vi "Teste.vi"() -> ()   [LabVIEW 2020]
uses:
  C:/Users/Opto/Downloads/GrabTestTDNI/GrabFrame2.dll
  Downloads/GrabTestTDNI/GrabFrame2.dll
  C:/Users/Opto/Desktop/Equipamentos/Teste/DALSA.SaperaLT.SapClassBasic.dll
  DALSA.SaperaLT.SapClassBasic.dll
panel:
  out "error SaveFrame":errorcluster
  out "error final":errorcluster
  out "error sapTransfer Dispose":errorcluster
  out "countFrame":i32
  out "Wait":bool
  out "Destroy":bool
  out "Create":bool
  out "framesArr":i16[][](array[numeric])
  out "Abriu arquivo?":bool
  out "filePath":string="C:\\temp\\IC-47_TDI.ccf"
  # "Buffer"
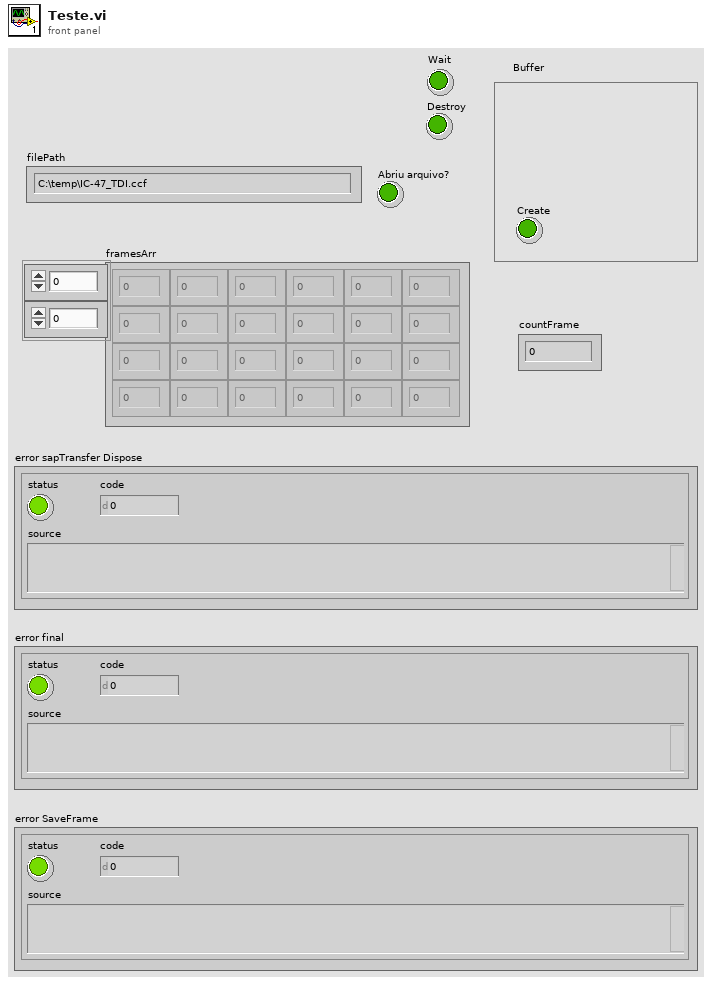
[diagram p1: front panel]
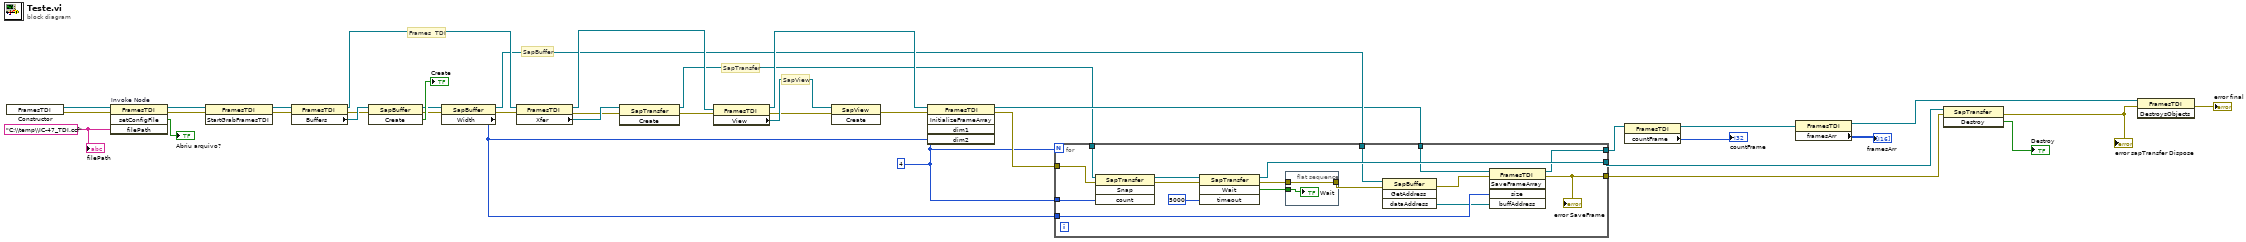
[diagram p0: block diagram]
diagram:
  w13 = 4 ("count")
  w35 = "C:\\temp\\IC-47_TDI.ccf" ("filePath")
  # "SapView"
  # "SapTransfer"
  # "SapBuffer"
  # "Frames  TDI"
  n1 = constructor class="FramesTDI"() -> (reference out=w38:refnum<k24>, error out=w39:errorcluster)  [unwired: 3 in, 1 out]
  n2 = invoke on="Invoke Node" class="FramesTDI" method="setConfigFile"(reference=w38, error in=w39, "filePath"=w35) -> (reference out=w37:refnum<k24>, error out=w36:errorcluster, "setConfigFile"=→"Abriu arquivo?":bool)  [unwired: 1 in, 1 out]
  n3 = invoke class="FramesTDI" method="StartGrabFramesTDI"(reference=w37, error in=w36) -> (reference out=w33:refnum<k24>, error out=w27:errorcluster)  [unwired: 1 in, 1 out]
  n4 = property class="FramesTDI"(reference=w33, error in=w27) -> (reference out=w20:refnum<k24>, error out=w26:errorcluster, "Buffers"=w32:refnum<k24>)
  n5 = invoke class="SapBuffer" method="Create"(reference=w32, error in=w26) -> (reference out=w28:refnum<k24>, error out=w25:errorcluster, "Create"=→"Create":bool)  [unwired: 1 in]
  n6 = property class="SapBuffer"(reference=w28, error in=w25) -> (reference out=w11:refnum<k24>, error out=w24:errorcluster, "Width"=w9:i32)
  n7 = property class="FramesTDI"(reference=w20, error in=w24) -> (reference out=w18:refnum<k24>, error out=w23:errorcluster, "Xfer"=w31:refnum<k24>)
  n8 = invoke class="SapTransfer" method="Create"(reference=w31, error in=w23) -> (reference out=w4:refnum<k24>, error out=w22:errorcluster)  [unwired: 1 in, 1 out]
  n9 = property class="FramesTDI"(reference=w18, error in=w22) -> (reference out=w17:refnum<k24>, error out=w21:errorcluster, "View"=w30:refnum<k24>)
  n10 = invoke class="SapView" method="Create"(reference=w30, error in=w21) -> (error out=w19:errorcluster)  [unwired: 1 in, 2 out]
  n11 = invoke class="FramesTDI" method="InitializeFrameArray"(reference=w17, error in=w19, "dim1"=w13, "dim2"=w9) -> (reference out=w10:refnum<k24>, error out=w14:errorcluster)  [unwired: 1 in, 3 out]
  n12 = for {
    N: w13 -> [_]
    tunnel: w4 -> [w56]
    tunnel: w14 -> [w55]
    tunnel: w13 -> [w54]
    tunnel: [w51] -> w12
    tunnel: w11 -> [w47]
    tunnel: w10 -> [w45]
    tunnel: w9 -> [w43]
    tunnel: [w41] -> w6
    tunnel: [w40] -> w8
    n13 = invoke class="SapTransfer" method="Snap"(reference=w56, error in=w55, "count"=w54) -> (reference out=w53:refnum<k24>, error out=w52:errorcluster)  [unwired: 1 in, 2 out]
    n14 = invoke class="SapTransfer" method="Wait"(reference=w53, error in=w52, "timeout"=5000) -> (reference out=w51:refnum<k24>, error out=w48:errorcluster, "Wait"=w49:bool)  [unwired: 1 in, 1 out]
    n15 = flat-sequence {
      tunnel: w49 -> [w58]
      tunnel: w48 -> [w57]
      tunnel: [w57] -> w46
      frame #0 {
        "Wait" <- w58
      }
    }
    n16 = invoke class="SapBuffer" method="GetAddress"(reference=w47, error in=w46) -> (error out=w44:errorcluster, "dataAddress"=w42:refnum<k24>)  [unwired: 2 in, 2 out]
    n17 = invoke class="FramesTDI" method="SaveFrameArray"(reference=w45, error in=w44, "size"=w43, "buffAddress"=w42) -> (reference out=w41:refnum<k24>, error out=w40:errorcluster)  [unwired: 1 in, 3 out]
    "error SaveFrame" <- w40
  }
  n18 = property class="FramesTDI"(reference=w6) -> (reference out=w7:refnum<k24>, "countFrame"=→"countFrame":i32)  [unwired: 1 in, 1 out]
  n19 = property class="FramesTDI"(reference=w7) -> (reference out=w3:refnum<k24>, "framesArr"=→"framesArr":i16[][])  [unwired: 1 in, 1 out]
  n20 = invoke class="SapTransfer" method="Destroy"(reference=w12, error in=w8) -> (error out=w1:errorcluster, "Destroy"=→"Destroy":bool)  [unwired: 1 in, 1 out]
  "error sapTransfer Dispose" <- w1
  n21 = invoke class="FramesTDI" method="DestroysObjects"(reference=w3, error in=w1) -> (error out=→"error final":errorcluster)  [unwired: 1 in, 2 out]
  "filePath" <- w35
